vi "Update Tag Double (Waveform).vi"(8 "error in (no error)":errorcluster, 9 "Waveform":waveform(dbl), 11 "Logger in.lvclass":refnum<class "Logger.lvclass">) -> (0 "error out":errorcluster, 3 "Logger out.lvclass":refnum<class "Logger.lvclass">)   [LabVIEW 2021, in "Logger.lvclass"]
uses:
  Logger.lvclass
  Logger.lvclass/Logger.ctl
  <vilib>/Skyline/Tag/Wrapper/Wrapper_class/Generate Tag Cluster (DBL) 2.vi
  <vilib>/Skyline/Tag/Shared/Serialize Double to String.vi
  <vilib>/Skyline/Tag/Wrapper/Wrapper_class/Generate Tag Cluster Core 2.vi
  <vilib>/Skyline/Tag/Wrapper/Wrapper_class/NI Skyline Tag.lvclass
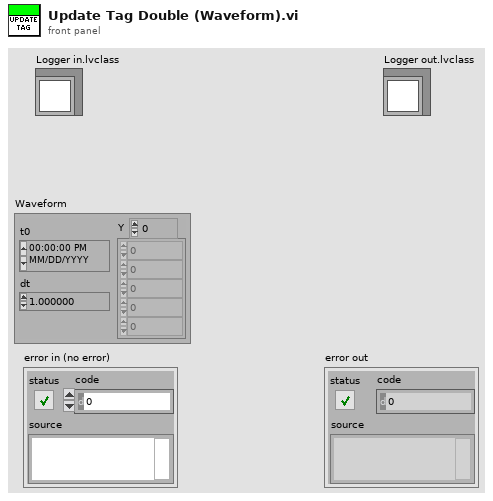
[diagram p1: front panel]
types:
  T1 = cluster{"Tag Units":string, "Tag Path":string, "Tag Reference":refnum<class "NI Skyline Tag.lvclass">}[]
  T2 = typedef "NI Skyline Tag.lvclass/Tag Value Cluster Wrapper.ctl" = cluster{"Configuration":refnum<class "NI Skyline Configuration.lvclass">, "Tag Cluster":T3}
  T3 = typedef "NI Skyline Tag.lvlib/Tag Value Cluster.ctl" = cluster{"Path":string, "Workspace ID":string, "Data Type":T4, "Value":string, "Time Stamp":timestamp}
  T4 = typedef "NI Skyline Tag.lvlib/DataType.ctl" = enum32{"Double", "I32", "String", "Boolean", "U64", "Timestamp"}
  T5 = cluster{"Tag Units":string, "Tag Path":string, "Tag Reference":refnum<class "NI Skyline Tag.lvclass">}
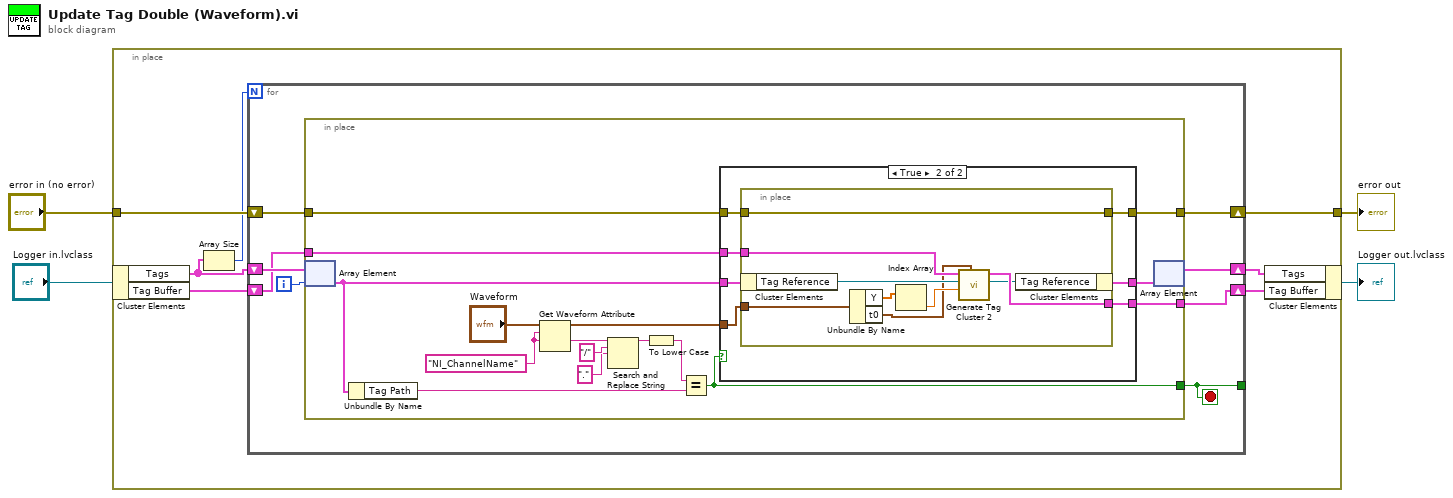
[diagram p0: block diagram]
diagram:
  n1 = in-place {
    in-place-border: "error in (no error)" -> [w10]
    in-place-border: [w9] -> w1
    n2 = in-place-cluster #1("Logger in.lvclass") -> ("Tags"=w7:T1, "Tag Buffer"=w6:T2[])
    n3 = Array Size(array=w7) -> (size(s)=w8:i32)
    n4 = for {
      N: w8 -> [_]
      shift-right: [w17] -> w11
      shift-left: w7 -> [w19]
      shift-right: [w15] -> w9
      shift-left: w10 -> [w16]
      shift-right: [w13] -> w5
      shift-left: w6 -> [w14]
      tunnel: [w12] -> _
      i -> [w18]
      stop <- w12 stop-if-true
      n5 = in-place {
        in-place-border: [w30] -> w12
        in-place-border: w16 -> [w33]
        in-place-border: [w32] -> w15
        in-place-border: w14 -> [w29]
        in-place-border: [w28] -> w13
        w27 = "NI_ChannelName" ("name")
        n6 = in-place-array #2(w19, w18) -> (w34:T5)
        n7 = Unbundle By Name(w34) -> ("Tag Path"=w31:string)
        n8 = Get Waveform Attribute(5:w27, 6:w27, 7:"Waveform") -> (1:w24:string, 3:w25:waveform(dbl))  [unwired: 1 in, 2 out]
        n9 = Search and Replace String(input string=w24, search string="/", replace string="." ("search string")) -> (result string=w21:string)  [unwired: 5 in, 3 out]
        n10 = To Lower Case(string=w21) -> (all lower case string=w20:string)
        n11 = Equal?(x=w20, y=w31) -> (x = y?=w30:bool)
        n12 = case shown="True" w30 {
          tunnel: w34 -> [w38 w45]
          tunnel: [w38 w44] -> w35
          tunnel: w33 -> [w37 w43]
          tunnel: [w37 w41] -> w32
          tunnel: w29 -> [w36 w42]
          tunnel: [w36 w40] -> w28
          tunnel: w25 -> [_ w39]
          frame False {
          }
          frame True {
            n13 = in-place {
              in-place-border: w43 -> [w54]
              in-place-border: w42 -> [w52]
              in-place-border: [w54] -> w41
              in-place-border: [w51] -> w40
              in-place-border: w39 -> [w49]
              n14 = in-place-cluster #3(w45) -> ("Tag Reference"=w53:refnum<class "NI Skyline Tag.lvclass">)
              n15 = Unbundle By Name(w49) -> ("Y"=w48:dbl[], "t0"=w46:timestamp)
              n16 = Index Array(array=w48) -> (element=w47:dbl)  [unwired: 1 in]
              n17 = call-poly <vilib>:"Generate Tag Cluster 2.vi"("time stamp"=w46, "value"=w47, "tag in"=w53, "tag clusters in"=w52) -> ("tag out"=w50:refnum<class "NI Skyline Tag.lvclass">, "tag clusters out"=w51:T2[])  [unwired: 5 in, 1 out]
              n18 = in-place-cluster #3("Tag Reference"=w50) -> (w44:T5)
            }
          }
        }
        n19 = in-place-array #2(w35) -> (w17:T1)  [unwired: 1 out]
      }
    }
    n20 = in-place-cluster #1("Tags"=w11, "Tag Buffer"=w5) -> (→"Logger out.lvclass":refnum<class "Logger.lvclass">)
  }
  "error out" <- w1
